vi "Set Buffer Read Position.vi"(8 "error in (no error)":errorcluster, 10 "Buffer Command":T1, 11 "CIF_CIPC_Chn in":refnum<class "CIF_CIPC_Chn.lvclass">) -> (0 "error out":errorcluster)   [LabVIEW 2021, in "CIF_CIPC_Chn.lvclass"]
uses:
  CIF_CIPC_Chn.lvclass
  CIF_CIPC_Chn.lvclass/CIF_CIPC_Chn.ctl
  <vilib>/CIF Foundation/CIF CIPC/SubVIs/Check Error.vi
  <vilib>/CIF Foundation/CIF CIPC/SubVIs/Get dll Path.vi
  <vilib>/Utility/error.llb/Trim Whitespace.vi
  <vilib>/Utility/error.llb/Error Cluster From Error Code.vi
  <vilib>/CIF Foundation/CIF CIPC/CIF_NI_CIPC.lvlib
  <vilib>/CIF Foundation/CIF CIPC/TypeDefs/Read Position.ctl
  Typedef/Buffer Control.ctl
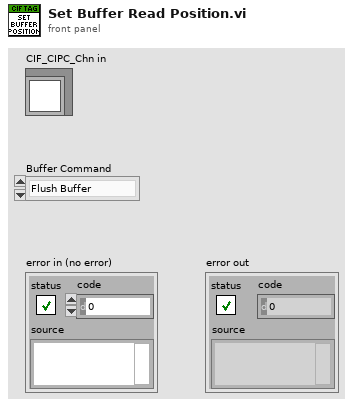
[diagram p1: front panel]
types:
  T1 = typedef "CIF_CIPC_Chn.lvclass/Buffer Control.ctl" = enum16{"Flush Buffer", "Newest Element", "Oldest Element"}
  T2 = typedef "CIF_NI_CIPC.lvlib/Read Position.ctl" = enum16{"Next", "Newest", "Oldest", "Next Available", "Absolute"}
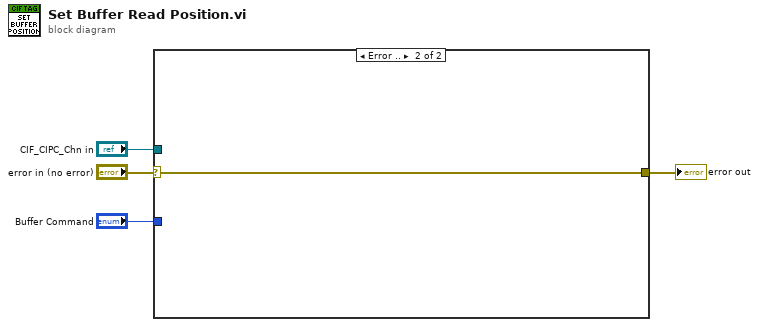
[diagram p0: block diagram]
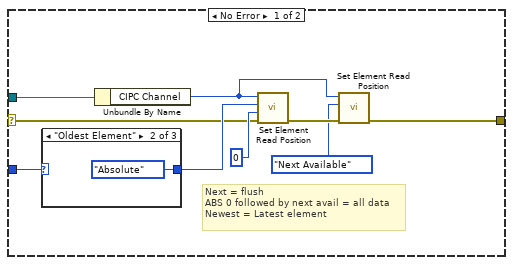
[diagram p2: hidden frame]
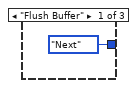
[diagram p3: hidden frame]
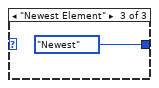
[diagram p4: hidden frame]
diagram:
  n1 = case shown="Error .." "error in (no error)" {
    selector: "error in (no error)" -> [w5 w17]
    tunnel: "CIF_CIPC_Chn in" -> [w13 _]
    tunnel: [w9 w17] -> w3
    tunnel: "Buffer Command" -> [w7 _]
    frame No Error {
      # "Next = flush\nABS 0 followed by next avail = all data\nNewest = Latest element"
      n2 = case shown="\"Oldest Element\"" w7 {
        tunnel: [Read_Position."Next" ("Read Position") Read_Position."Absolute" ("Read Position") Read_Position."Newest" ("Read Position")] -> w8
        frame "Flush Buffer" {
        }
        frame "Oldest Element" {
        }
        frame "Newest Element" {
        }
      }
      n3 = Unbundle By Name(w13) -> ("CIPC Channel"=w11:u64)
      n4 = call <vilib>:"Set Element Read Position.vi"("error in (no error)"=w5, "Element Index Offset"=0, "Read Position"=w8, "CIPC Reference"=w11) -> ("error out"=w10:errorcluster)  [unwired: 7 in]
      n5 = call <vilib>:"Set Element Read Position.vi"("error in (no error)"=w10, "Read Position"=Read_Position."Next Available", "CIPC Reference"=w11) -> ("error out"=w9:errorcluster)  [unwired: 8 in]
    }
    frame Error {
    }
  }
  "error out" <- w3
